vi "nominal workspace rid.vi"(7 "out_needed":u32, 8 "error in (no error)":errorcluster, 9 "cap":u32, 10 "buf":string, 11 "workspace":i32) -> (0 "error out":errorcluster, 2 "buf out":string, 3 "function return":i32, 5 "out_needed out":u32)   [LabVIEW 2020, in "client.lvlib"]
doc: "int32_t nominal_workspace_rid(int32_t workspace, char *buf, uint32_t cap, uint32_t *out_needed);"
uses:
  client.lvlib
  bin/nominalClient_64.dll
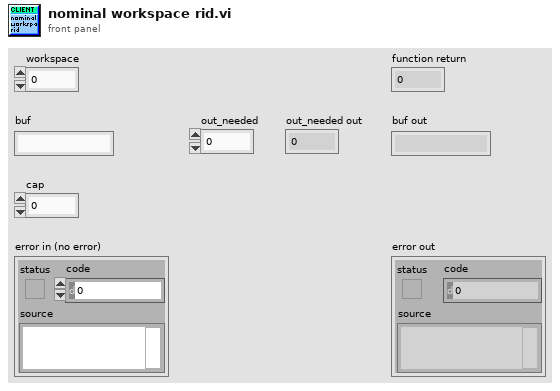
[diagram p1: front panel]
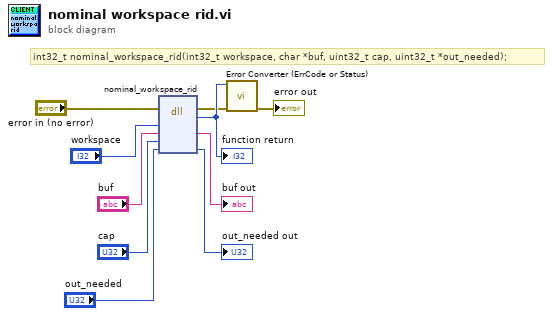
[diagram p0: block diagram]
diagram:
  # "int32_t nominal_workspace_rid(int32_t workspace, char *buf, uint32_t cap, uint32_t *out_needed);"
  n1 = dll-call lib="C:/code/labview-client-rs/lv_src/bin/nominalClient_*.*" fn="nominal_workspace_rid"(error in="error in (no error)", "workspace"="workspace", "buf"="buf", "cap"="cap", "out_needed"="out_needed") -> (error out=w2:errorcluster, w10:i32, "buf"=→"buf out":string, "out_needed"=→"out_needed out":u32)  [unwired: 4 in, 1 out]
  "function return" <- w10
  n2 = call "Error Converter (ErrCode or Status).vi"("error in (no error)"=w2, "error code"=w10) -> ("error out"=→"error out":errorcluster)  [unwired: 9 in]
